vi "+S2C_UNITHERM_Process.vi"(8 "Error In":errorcluster) -> (0 "Error Out":errorcluster)   [LabVIEW 2015]
uses:
  VIs/S2C_UNITHERM_Proc_Globals.vi
panel:
  out "Err":bool
  in  "Clear":bool
  out "Exit":bool
  in  "LogDepth":u32=10 caption="Log Depth"
  in  "CtrlTab":enum32{"UniTherm"}(tab)
  in  "P1":T1={"P1C1"={"Resource Name"="COM4", "Baud Rate"=57600, "Data Bits"=8, "Parity"=0, "Stop Bits"=10, "Flow Control"=0, "Termination Char"=10, "Enable Termination"=TRUE, "Timeout"=5000, "P1C1Exe"=FALSE}, "P1C2"={"UniCmd"=enum."Reset", "Numeric Return"="", "Manufacturer"="", "Model Number"="", "Serial Number"="", "Firmware Version"="", "Status"={"Active"=FALSE, "Protected"=FALSE, "Disconnected"=FALSE}, "P1C2Exe"=FALSE}, "P1C3"={"Load Impedance"=100, "P1C3Exe"=FALSE}, "P1C4"={"Command"="*IDN?", "Action"="READ", "P1C4Exe"=FALSE}} {"P1C1"."Parity" items=["None", "Odd", "Even", "Mark", "Space"]; "P1C1"."Flow Control" items=["None", "XON/XOFF", "RTS/CTS", "XON/XOFF & RTS/CTS", "DTR/DSR", "XON/XOFF & DTR/DSR"]; "P1C1"."Stop Bits" items=["1.0"=10, "1.5"=15, "2.0"=20]; "P1C1"."Data Bits" min=5 max=8 step=1}
  in  "CommLog":string caption="Communication Log"
  # "Main Cluster:\n394x886\n1 = 355x876\n2 = 355x438\n3 = 355x292\n4 = 163x438\n6 = 163x292\n8 = 163x219"
  # "UniTherm Driver Panel"
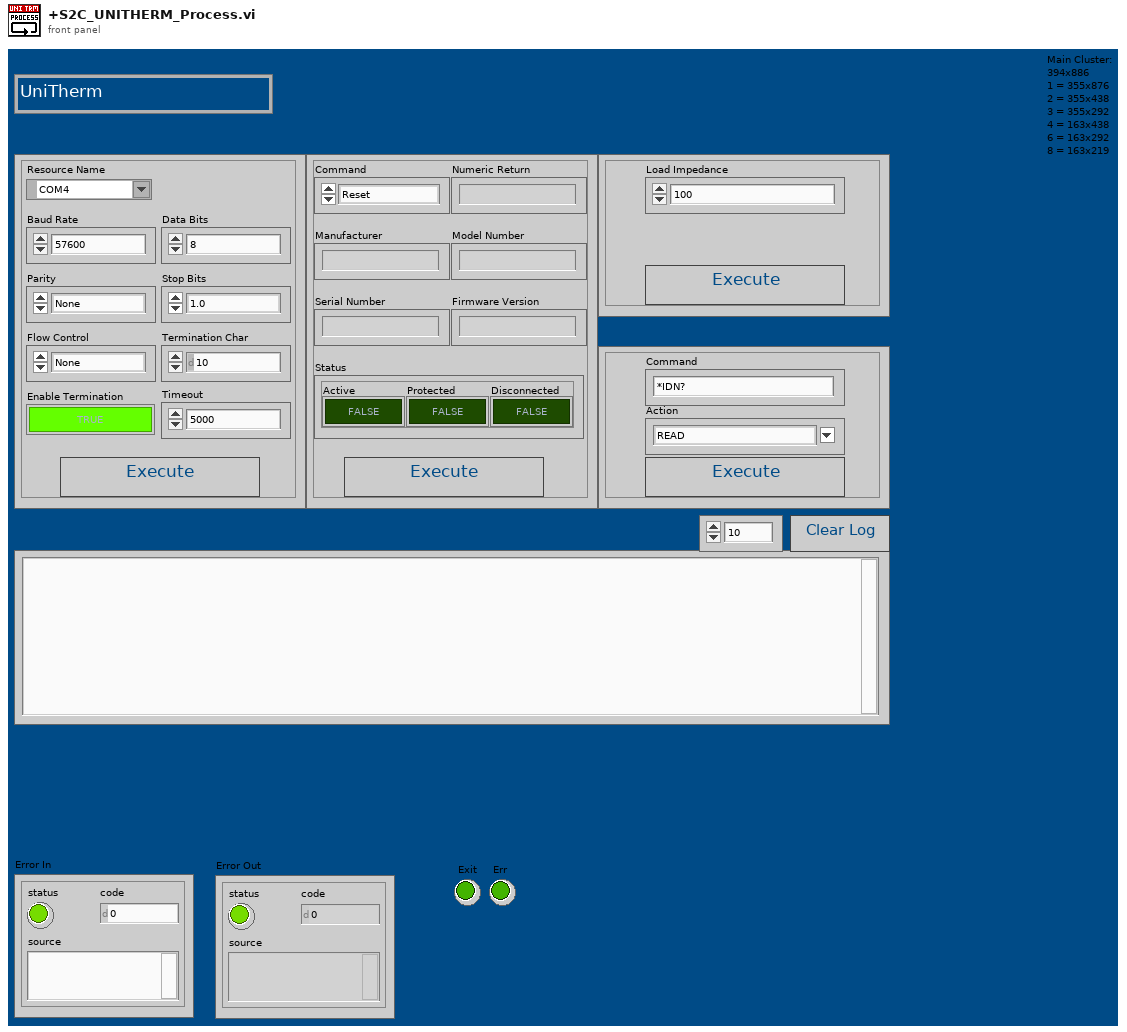
[diagram p1: front panel]
types:
  T1 = cluster{"P1C1":cluster{"Resource Name":refnum<visa-resource-name>, "Baud Rate":u32, "Data Bits":u16, "Parity":u16, "Stop Bits":u16, "Flow Control":u16, "Termination Char":u8, "Enable Termination":bool, "Timeout":u32, "P1C1Exe":bool}, "P1C2":cluster{"UniCmd":enum16{"Reset", "Status", "Identify", "SelfTest", "Protection On", "Protection Off", "Load Clear", "Crest Factor", "RMS Current", "Peak Current", "RMS Voltage", "Peak Voltage"}, "Numeric Return":string, "Manufacturer":string, "Model Number":string, "Serial Number":string, "Firmware Version":string, "Status":cluster{"Active":bool, "Protected":bool, "Disconnected":bool}, "P1C2Exe":bool}, "P1C3":cluster{"Load Impedance":i32, "P1C3Exe":bool}, "P1C4":cluster{"Command":string, "Action":string, "P1C4Exe":bool}}
  T2 = cluster{"Caller-Q":refnum<queue>, "Command":string, "Return":string, "Data":variant, "Timeout":dbl}
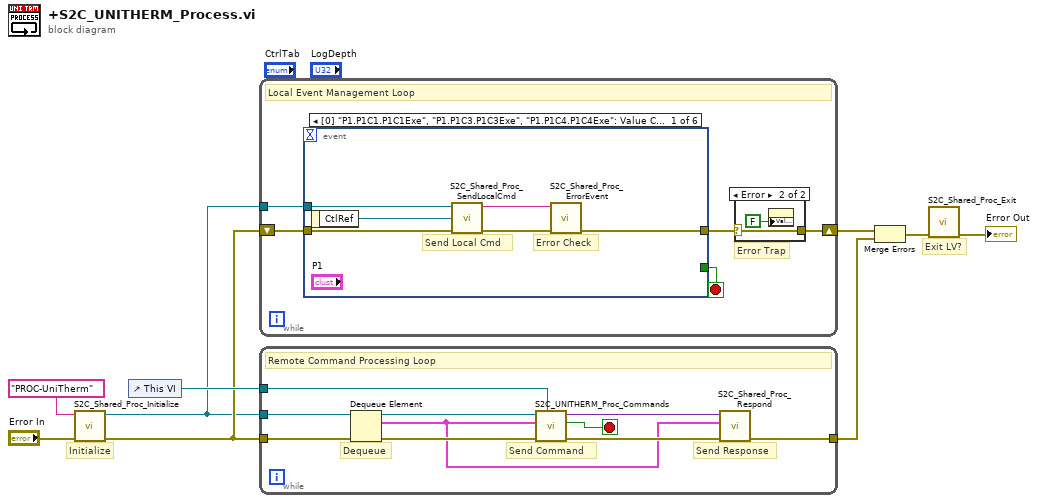
[diagram p0: block diagram]
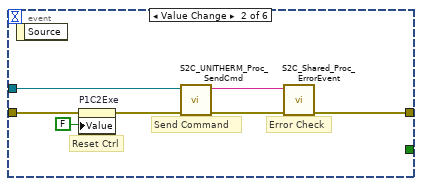
[diagram p3: hidden frame]
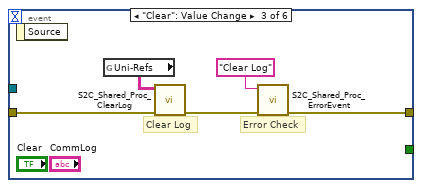
[diagram p4: hidden frame]
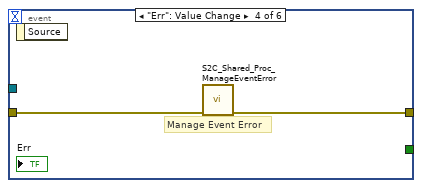
[diagram p5: hidden frame]
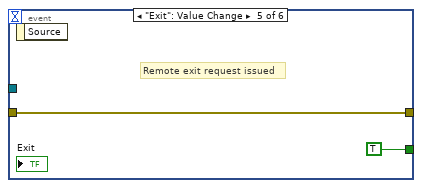
[diagram p6: hidden frame]
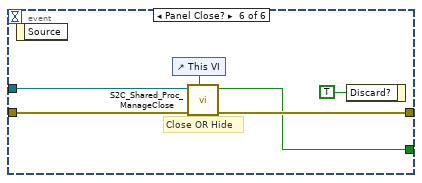
[diagram p7: hidden frame]
diagram:
  # "Exit LV?"
  # "Initialize"
  n1 = call "S2C_Shared_Proc_Initialize.vi"("Error In"="Error In", "Q-Name"="PROC-UniTherm" ("name (unnamed)")) -> ("Error Out"=w4:errorcluster, "Q-Ref"=w1:refnum<queue>)  [unwired: 8 in]
  n2 = control-ref of="This VI"() -> (w5:refnum<vi>)
  n3 = while {
    tunnel: w1 -> [w13]
    shift-right: [w10] -> w7
    shift-left: w4 -> [w14]
    stop <- w12 stop-if-true
    # "Error Trap"
    # "Local Event Management Loop"
    n4 = event shown="[0] \"P1.P1C1.P1C1Exe\", \"P1.P1C3.P1C3Exe\", \"P1.P1C4.P1C4Exe\": Value Change" {
      selector: _ -> [_ _ _ _ _ _]
      dyn-events: _ -> [_ _ _ _ _ _]
      timeout: _ -> [_ _ _ _ _ _]
      tunnel: w14 -> [w23 w29 w35 w37 w39 w44]
      tunnel: w13 -> [w22 w30 _ _ _ w42]
      tunnel: [w19 w24 w32 w36 w39 w43] -> w11
      tunnel: [_ _ _ _ TRUE ("Discard?") w41] -> w12
      event "P1.P1C1.P1C1Exe", "P1.P1C3.P1C3Exe", "P1.P1C4.P1C4Exe": Value Change {
        # "Error Check"
        # "Send Local Cmd"
        n5 = event-data() -> ("CtlRef"=w21:refnum<vi>)  [unwired: 1 in]
        n6 = call "S2C_Shared_Proc_SendLocalCmd.vi"("Error In"=w23, "ExeRef"=w21, "Q-Ref"=w22) -> ("Error Out"=w20:errorcluster, "Command"=w18:string)  [unwired: 7 in]
        n7 = call "S2C_Shared_Proc_ErrorEvent.vi"("Error In"=w20, "Command"=w18) -> ("Error Out"=w19:errorcluster)  [unwired: 9 in]
      }
      event "P1.P1C2.P1C2Exe": Value Change {
        # "Error Check"
        # "Reset Ctrl"
        # "Send Command"
        n8 = event-data() -> ()  [unwired: 1 in, 1 out]
        n9 = property on="P1C2Exe" class="Bool (strict)"(error in=w29, "Value"=FALSE) -> (error out=w28:errorcluster)  [unwired: 1 in, 1 out]
        n10 = call "S2C_UNITHERM_Proc_SendCmd.vi"("Error In"=w28, "Q-Ref"=w30) -> ("Error Out"=w26:errorcluster, "Command"=w25:string)  [unwired: 8 in]
        n11 = call "S2C_Shared_Proc_ErrorEvent.vi"("Error In"=w26, "Command"=w25) -> ("Error Out"=w24:errorcluster)  [unwired: 9 in]
      }
      event "Clear": Value Change {
        # "Error Check"
        # "Clear Log"
        n12 = event-data() -> ()  [unwired: 1 in, 1 out]
        n13 = global read "S2C_UNITHERM_Proc_Globals.vi" "Uni-Refs"() -> (w33:string[][])
        n14 = call "S2C_Shared_Proc_ClearLog.vi"("Error In"=w35, "Refs"=w33) -> ("Error Out"=w34:errorcluster)  [unwired: 9 in]
        n15 = call "S2C_Shared_Proc_ErrorEvent.vi"("Error In"=w34, "Command"="Clear Log") -> ("Error Out"=w32:errorcluster)  [unwired: 9 in]
      }
      event "Err": Value Change {
        # "Manage Event Error"
        n16 = event-data() -> ()  [unwired: 1 in, 1 out]
        n17 = call "S2C_Shared_Proc_ManageEventError.vi"("Error In"=w37) -> ("Error Out"=w36:errorcluster)  [unwired: 10 in]
      }
      event "Exit": Value Change {
        # "Remote exit request issued"
        n18 = event-data() -> ()  [unwired: 1 in, 1 out]
      }
      event Panel Close? {
        # "Close OR Hide"
        n19 = event-data() -> ()  [unwired: 1 in, 1 out]
        n20 = control-ref of="This VI"() -> (w40:refnum<vi>)
        n21 = call "S2C_Shared_Proc_ManageClose.vi"("VI_Ref"=w40, "Error In"=w44, "Q-Ref"=w42) -> ("Error Out"=w43:errorcluster, "Exit?"=w41:bool)  [unwired: 7 in]
        n22 = event-data("Discard?"=TRUE) -> ()  [unwired: 1 in, 1 out]
      }
    }
    n23 = case shown="Error" w11 {
      selector: w11 -> [w15 w17]
      tunnel: [w15 w17] -> w10
      frame No Error {
      }
      frame Error {
        n24 = property on="Err" class="Bool (strict)"("Val(Sgnl)"=FALSE ("Value (Signaling)")) -> ()  [unwired: 2 in, 2 out]
      }
    }
  }
  n25 = while {
    tunnel: w1 -> [w46]
    tunnel: w5 -> [w50]
    tunnel: w4 -> [w55]
    tunnel: [w49] -> w6
    stop <- w51 stop-if-true
    # "Send Response"
    # "Send Command"
    # "Dequeue"
    # "Remote Command Processing Loop"
    n26 = Dequeue Element(queue=w46, error in (no error)=w55) -> (queue out=w48:refnum<queue>, element=w47:T2, error out=w54:errorcluster)  [unwired: 1 in, 1 out]
    n27 = call "S2C_UNITHERM_Proc_Commands.vi"("VI_Ref"=w50, "Error In"=w54, "Settings"=w47, "Q-Ref"=w48) -> ("Error Out"=w52:errorcluster, "Stop?"=w51:bool, "Response"=w53:variant)  [unwired: 5 in]
    n28 = call "S2C_Shared_Proc_Respond.vi"("Error In"=w52, "Settings"=w47, "Response"=w53) -> ("Error Out"=w49:errorcluster)  [unwired: 8 in]
  }
  n29 = Merge Errors(w7, w6) -> (w3:errorcluster)
  n30 = call "S2C_Shared_Proc_Exit.vi"("Error In"=w3) -> ("Error Out"=→"Error Out":errorcluster)  [unwired: 10 in]
